vi "Eurotherm_Hardware_Module.vi"(3 "SP":bool=TRUE, 4 "Decimales":u16(ring)=1 items=["0"=1, "1"=10, "2"=100], 5 "Eurotherm (T:Enable)":bool=TRUE, 7 "Command":T2, 8 "error in (no error)":errorcluster, 9 "Value":dbl format="%04.1g", 10 "Address":T1(ring), 11 "VISA resource name":refnum<visa-resource-name>) -> (0 "error out":errorcluster, 1 "PV(C)":dbl, 2 "SP(C)":dbl)   [LabVIEW 2013]
uses:
  Eurotherm_Hardware_Module Control.ctl
  <vilib>/Instr/_visa.llb/VISA Configure Serial Port (Instr).vi
panel:
  out "String Read":string
  out "String Write":string
  # "Input Data"
  # "Local Data"
  # "Output Data"
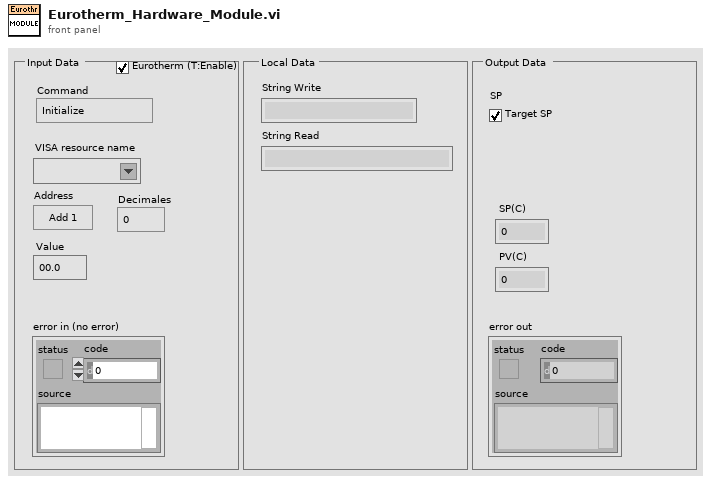
[diagram p1: front panel]
types:
  T1 = enum16{"Add 1", "Add 2", "Add 10", "Add 11", "Add 12", "Add 13"}
  T2 = typedef "Eurotherm_Hardware_Module Control.ctl" = enum16{"Initialize", "Write SP", "Read SP+PV", "Write Rate", "Set P", "Set I", "Set D", "Shutdown"}
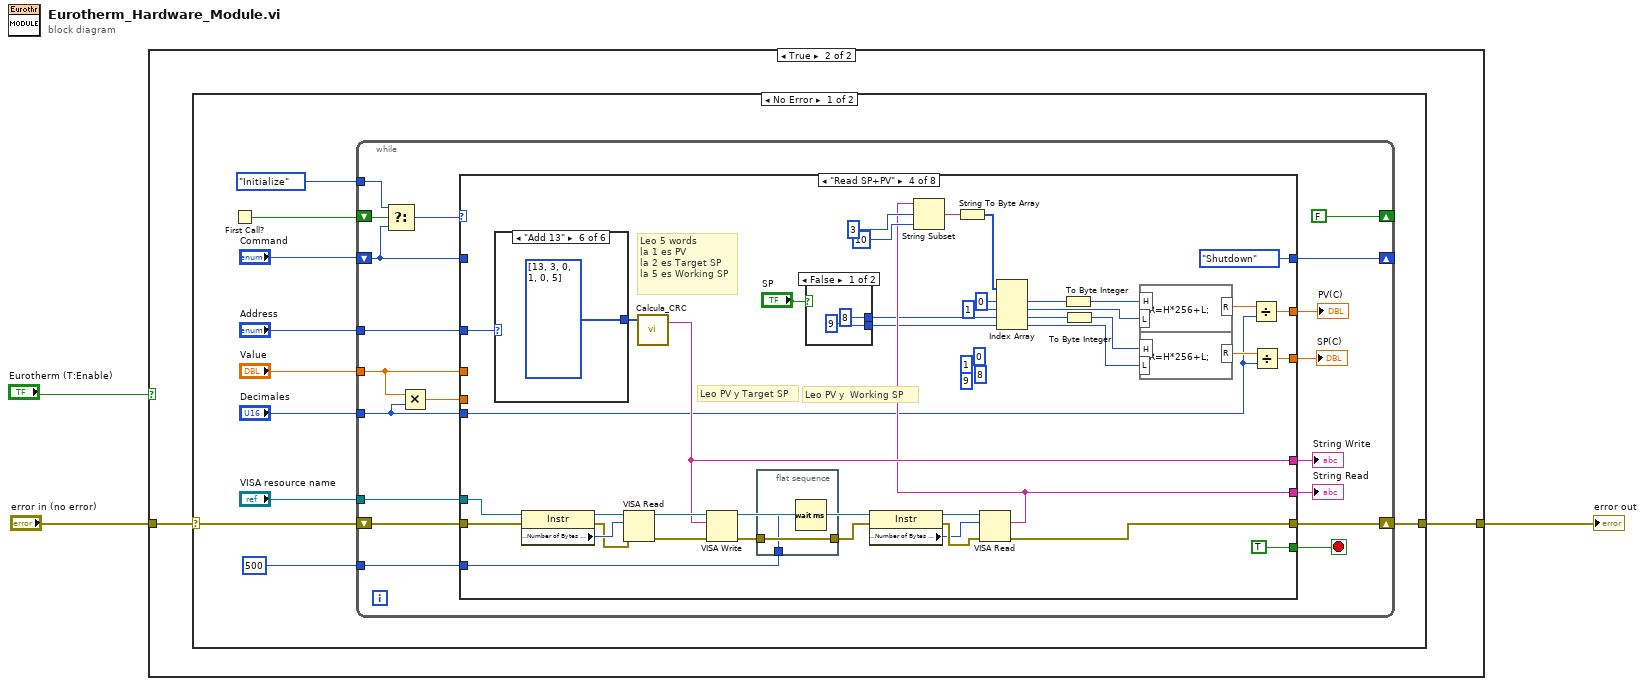
[diagram p0: block diagram]
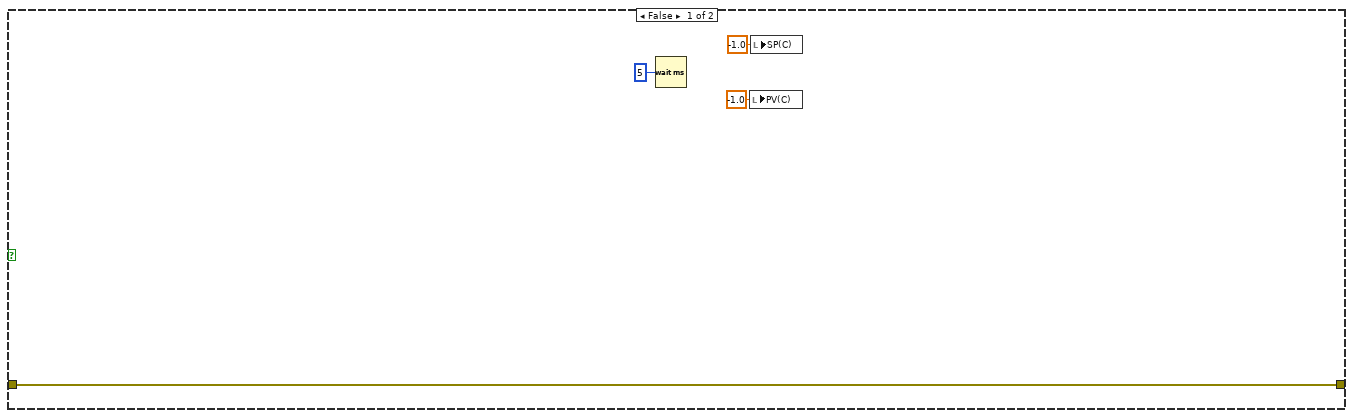
[diagram p2: hidden frame]
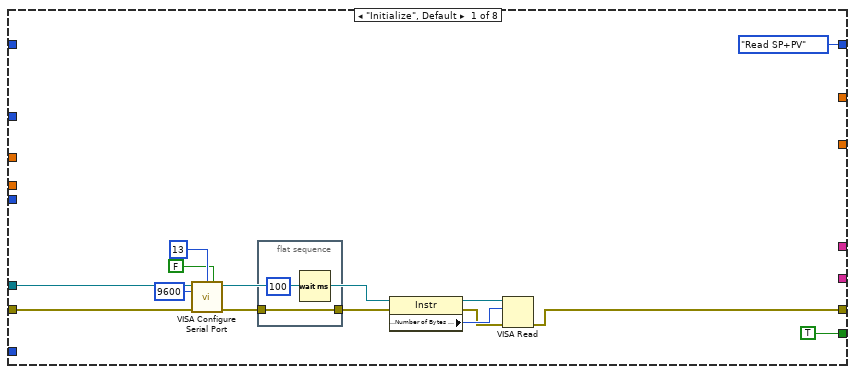
[diagram p3: hidden frame]
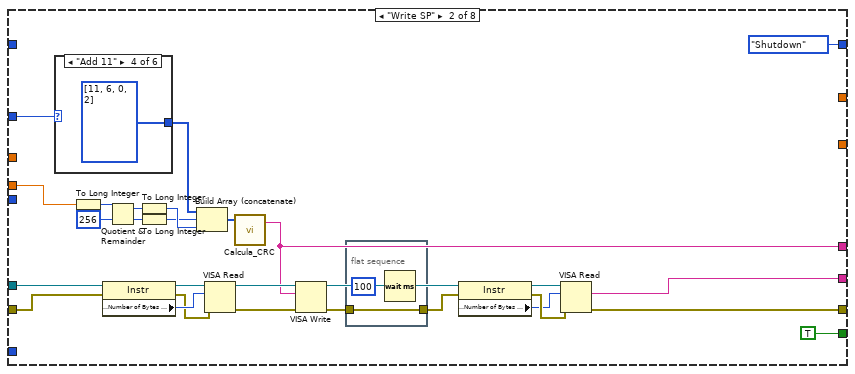
[diagram p4: hidden frame]
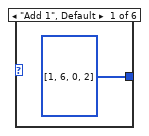
[diagram p5: hidden frame]
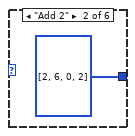
[diagram p6: hidden frame]
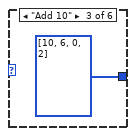
[diagram p7: hidden frame]
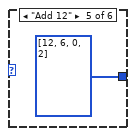
[diagram p8: hidden frame]
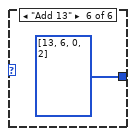
[diagram p9: hidden frame]
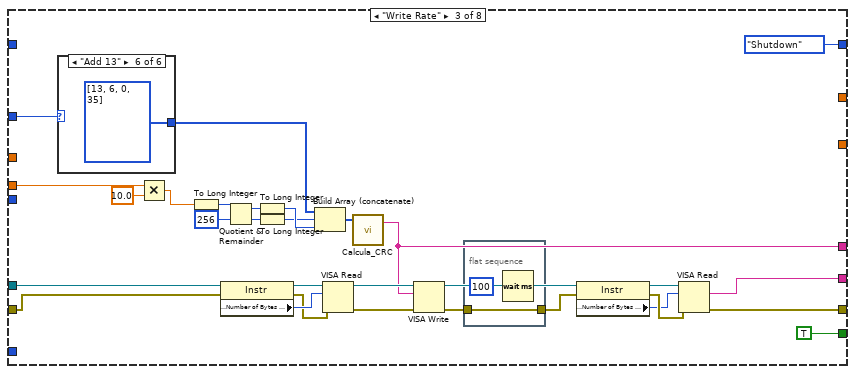
[diagram p10: hidden frame]
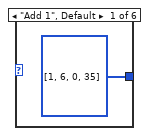
[diagram p11: hidden frame]
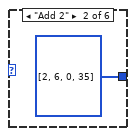
[diagram p12: hidden frame]
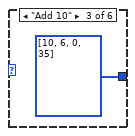
[diagram p13: hidden frame]
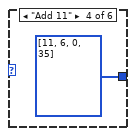
[diagram p14: hidden frame]
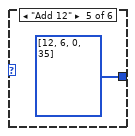
[diagram p15: hidden frame]
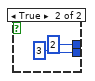
[diagram p16: hidden frame]
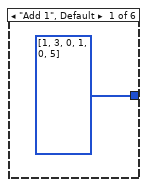
[diagram p17: hidden frame]
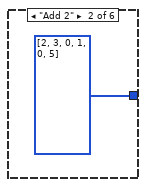
[diagram p18: hidden frame]
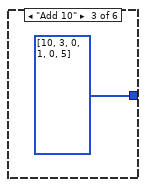
[diagram p19: hidden frame]
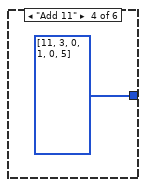
[diagram p20: hidden frame]
diagram:
  n1 = case shown="True" "Eurotherm (T:Enable)" {
    tunnel: "error in (no error)" -> [w7 w9]
    tunnel: [w7 w8] -> w2
    frame False {
      n2 = Wait (ms)(milliseconds to wait=u32 5) -> ()  [unwired: 1 out]
      n3 = local write "PV(C)"(-1.0 ("PV(C)")) -> ()
      n4 = local write "SP(C)"(-1.0 ("SP(C)")) -> ()
    }
    frame True {
      n5 = case shown="No Error" w9 {
        selector: w9 -> [w17 w295]
        tunnel: [w16 w295] -> w8
        frame No Error {
          n6 = First Call?() -> (First Call?: T/F=w19:bool)
          n7 = while {
            shift-right: [w33] -> _
            shift-left: "Command" -> [w34]
            shift-right: [w31] -> w16
            shift-left: w17 -> [w30]
            shift-right: [FALSE ("First Call?: T/F")] -> _
            shift-left: w19 -> [w38]
            tunnel: Eurotherm_Hardware_Module_Control."Initialize" ("t") -> [w37]
            tunnel: "Address" -> [w27]
            tunnel: "Value" -> [w22]
            tunnel: "Decimales" -> [w24]
            tunnel: "VISA resource name" -> [w21]
            tunnel: u32 500 ("milliseconds to wait") -> [w20]
            stop <- w32 stop-if-true
            n8 = Select(t=w37, s=w38, f=w34) -> (s? t:f=w35:T2)
            n9 = Multiply(x=w22, y=w24) -> (x*y=w23:dbl)
            n10 = case shown="\"Read SP+PV\"" w35 {
              tunnel: w34 -> [_ _ _ _ _ _ _ _]
              tunnel: [Eurotherm_Hardware_Module_Control."Read SP+PV" ("s? t:f") Eurotherm_Hardware_Module_Control."Shutdown" ("s? t:f") Eurotherm_Hardware_Module_Control."Shutdown" ("s? t:f") Eurotherm_Hardware_Module_Control."Shutdown" ("s? t:f") Eurotherm_Hardware_Module_Control."Shutdown" ("s? t:f") Eurotherm_Hardware_Module_Control."Shutdown" ("s? t:f") Eurotherm_Hardware_Module_Control."Shutdown" ("s? t:f") Eurotherm_Hardware_Module_Control."Shutdown" ("s? t:f")] -> w33
              tunnel: [TRUE ("First Call?: T/F") TRUE ("First Call?: T/F") TRUE ("First Call?: T/F") TRUE ("First Call?: T/F") TRUE ("First Call?: T/F") TRUE ("First Call?: T/F") TRUE ("First Call?: T/F") TRUE ("First Call?: T/F")] -> w32
              tunnel: [w42 w62 w96 w140 w189 w225 w261 w290] -> w31
              tunnel: w30 -> [w43 w63 w100 w156 w190 w226 w262 w291]
              tunnel: w21 -> [w39 w61 w101 w155 w188 w224 w260 w292]
              tunnel: [_ w60 w95 w141 w187 w223 w259 _] -> w29
              tunnel: [_ w59 w94 w154 w186 w222 w258 _] -> w28
              tunnel: w27 -> [_ w56 w99 w169 w183 w219 w255 _]
              tunnel: [_ _ _ w136 _ _ _ _] -> w26
              tunnel: [_ _ _ w135 _ _ _ _] -> w25
              tunnel: w23 -> [_ w55 w93 _ _ _ _ _]
              tunnel: w24 -> [_ _ _ w137 _ _ _ _]
              tunnel: w22 -> [_ _ _ _ w182 w218 w254 _]
              tunnel: w20 -> [_ _ _ w132 _ _ _ _]
              frame "Initialize", Default {
                n11 = call-poly "VISA Configure Serial Port"("VISA resource name"=w39, "termination char\n(0xA = '\\n' = LF)"=u8 13 ("termination char\n(0xA = '\\n' = LF)"), "Enable Termination\nChar (T)"=FALSE ("Enable Termination\nChar (T)"), "baud rate (9600)"=u32 9600, "error in (no error)"=w43) -> ("VISA resource name out"=w44:refnum<visa-resource-name>, "error out"=w45:errorcluster)  [unwired: 9 in]
                n12 = flat-sequence {
                  tunnel: w45 -> [w53]
                  tunnel: [w53] -> w52
                  frame #0 {
                    n13 = Wait (ms)(milliseconds to wait=u32 100) -> ()  [unwired: 1 out]
                  }
                }
                n14 = property class="Instr"(reference=w44, error in=w52) -> (reference out=w49:refnum<visa-resource-name>, error out=w50:errorcluster, "Serial Settings:Number of Bytes at Serial Port"=w51:u32)
                n15 = VISA Read(VISA resource name=w49, byte count=w51, error in (no error)=w50) -> (error out=w42:errorcluster)  [unwired: 3 out]
              }
              frame "Write SP" {
                n16 = case shown="\"Add 11\"" w56 {
                  tunnel: [u8[] [1, 6, 0, 2] ("Message Data") u8[] [2, 6, 0, 2] ("Message Data") u8[] [10, 6, 0, 2] ("Message Data") u8[] [11, 6, 0, 2] ("Message Data") u8[] [12, 6, 0, 2] ("Message Data") u8[] [13, 6, 0, 2] ("Message Data")] -> w82
                  frame "Add 1", Default {
                  }
                  frame "Add 2" {
                  }
                  frame "Add 10" {
                  }
                  frame "Add 11" {
                  }
                  frame "Add 12" {
                  }
                  frame "Add 13" {
                  }
                }
                n17 = To Long Integer(number=w55) -> (32bit integer=w81:i32)
                n18 = property class="Instr"(reference=w61, error in=w63) -> (reference out=w64:refnum<visa-resource-name>, error out=w65:errorcluster, "Serial Settings:Number of Bytes at Serial Port"=w66:u32)
                n19 = Quotient & Remainder(x=w81, y=256) -> (x-y*floor(x/y)=w76:i32, floor(x/y)=w77:i32)
                n20 = To Long Integer(number=w76) -> (32bit integer=w79:i32)
                n21 = To Long Integer(number=w77) -> (32bit integer=w78:i32)
                n22 = Build Array (concatenate)(w82, w78, w79) -> (w80:i32[])
                n23 = VISA Read(VISA resource name=w64, byte count=w66, error in (no error)=w65) -> (VISA resource name out=w73:refnum<visa-resource-name>, error out=w72:errorcluster)  [unwired: 2 out]
                n24 = call "Calcula_CRC.vi"("Message Data"=w80) -> ("String"=w59:string)  [unwired: 2 in, 1 out]
                n25 = VISA Write(VISA resource name=w73, write buffer=w59, error in (no error)=w72) -> (VISA resource name out=w74:refnum<visa-resource-name>, error out=w71:errorcluster)  [unwired: 1 out]
                n26 = flat-sequence {
                  tunnel: w71 -> [w83]
                  tunnel: [w83] -> w70
                  frame #0 {
                    n27 = Wait (ms)(milliseconds to wait=u32 100) -> ()  [unwired: 1 out]
                  }
                }
                n28 = property class="Instr"(reference=w74, error in=w70) -> (reference out=w69:refnum<visa-resource-name>, error out=w68:errorcluster, "Serial Settings:Number of Bytes at Serial Port"=w67:u32)
                n29 = VISA Read(VISA resource name=w69, byte count=w67, error in (no error)=w68) -> (read buffer=w60:string, error out=w62:errorcluster)  [unwired: 2 out]
              }
              frame "Write Rate" {
                n30 = case shown="\"Add 13\"" w99 {
                  tunnel: [u8[] [1, 6, 0, 35] ("Message Data") u8[] [2, 6, 0, 35] ("Message Data") u8[] [10, 6, 0, 35] ("Message Data") u8[] [11, 6, 0, 35] ("Message Data") u8[] [12, 6, 0, 35] ("Message Data") u8[] [13, 6, 0, 35] ("Message Data")] -> w120
                  frame "Add 1", Default {
                  }
                  frame "Add 2" {
                  }
                  frame "Add 10" {
                  }
                  frame "Add 11" {
                  }
                  frame "Add 12" {
                  }
                  frame "Add 13" {
                  }
                }
                n31 = Multiply(x=w93, y=10.0) -> (x*y=w92:dbl)
                n32 = To Long Integer(number=w92) -> (32bit integer=w119:i32)
                n33 = property class="Instr"(reference=w101, error in=w100) -> (reference out=w102:refnum<visa-resource-name>, error out=w103:errorcluster, "Serial Settings:Number of Bytes at Serial Port"=w104:u32)
                n34 = Quotient & Remainder(x=w119, y=256) -> (x-y*floor(x/y)=w114:i32, floor(x/y)=w115:i32)
                n35 = To Long Integer(number=w114) -> (32bit integer=w117:i32)
                n36 = To Long Integer(number=w115) -> (32bit integer=w116:i32)
                n37 = Build Array (concatenate)(w120, w116, w117) -> (w118:i32[])
                n38 = VISA Read(VISA resource name=w102, byte count=w104, error in (no error)=w103) -> (VISA resource name out=w111:refnum<visa-resource-name>, error out=w110:errorcluster)  [unwired: 2 out]
                n39 = call "Calcula_CRC.vi"("Message Data"=w118) -> ("String"=w94:string)  [unwired: 2 in, 1 out]
                n40 = VISA Write(VISA resource name=w111, write buffer=w94, error in (no error)=w110) -> (VISA resource name out=w112:refnum<visa-resource-name>, error out=w109:errorcluster)  [unwired: 1 out]
                n41 = flat-sequence {
                  tunnel: w109 -> [w121]
                  tunnel: [w121] -> w108
                  frame #0 {
                    n42 = Wait (ms)(milliseconds to wait=u32 100) -> ()  [unwired: 1 out]
                  }
                }
                n43 = property class="Instr"(reference=w112, error in=w108) -> (reference out=w107:refnum<visa-resource-name>, error out=w106:errorcluster, "Serial Settings:Number of Bytes at Serial Port"=w105:u32)
                n44 = VISA Read(VISA resource name=w107, byte count=w105, error in (no error)=w106) -> (read buffer=w95:string, error out=w96:errorcluster)  [unwired: 2 out]
              }
              frame "Read SP+PV" {
                (unwired) 9 ("index")
                (unwired) 8 ("index")
                (unwired) 1 ("index")
                (unwired) 0 ("index")
                # "Leo PV y  Working SP"
                # "Leo PV y Target SP"
                # "Leo 5 words\nla 1 es PV\nla 2 es Target SP\nla 5 es Working SP"
                n45 = case shown="\"Add 13\"" w169 {
                  tunnel: [u8[] [1, 3, 0, 1, 0, 5] ("Message Data") u8[] [2, 3, 0, 1, 0, 5] ("Message Data") u8[] [10, 3, 0, 1, 0, 5] ("Message Data") u8[] [11, 3, 0, 1, 0, 5] ("Message Data") u8[] [12, 3, 0, 1, 0, 5] ("Message Data") u8[] [13, 3, 0, 1, 0, 5] ("Message Data")] -> w168
                  frame "Add 1", Default {
                  }
                  frame "Add 2" {
                  }
                  frame "Add 10" {
                  }
                  frame "Add 11" {
                  }
                  frame "Add 12" {
                  }
                  frame "Add 13" {
                  }
                }
                n46 = property class="Instr"(reference=w155, error in=w156) -> (reference out=w157:refnum<visa-resource-name>, error out=w158:errorcluster, "Serial Settings:Number of Bytes at Serial Port"=w159:u32)
                n47 = VISA Read(VISA resource name=w157, byte count=w159, error in (no error)=w158) -> (VISA resource name out=w166:refnum<visa-resource-name>, error out=w165:errorcluster)  [unwired: 2 out]
                n48 = call "Calcula_CRC.vi"("Message Data"=w168) -> ("String"=w154:string)  [unwired: 2 in, 1 out]
                n49 = VISA Write(VISA resource name=w166, write buffer=w154, error in (no error)=w165) -> (VISA resource name out=w167:refnum<visa-resource-name>, error out=w164:errorcluster)  [unwired: 1 out]
                n50 = flat-sequence {
                  tunnel: w164 -> [w175]
                  tunnel: [w175] -> w163
                  tunnel: w132 -> [w174]
                  frame #0 {
                    n51 = Wait (ms)(milliseconds to wait=w174) -> ()  [unwired: 1 out]
                  }
                }
                n52 = case shown="False" "SP" {
                  tunnel: [8 ("index") 2 ("index")] -> w130
                  tunnel: [9 ("index") 3 ("index")] -> w129
                  frame False {
                  }
                  frame True {
                  }
                }
                n53 = property class="Instr"(reference=w167, error in=w163) -> (reference out=w162:refnum<visa-resource-name>, error out=w161:errorcluster, "Serial Settings:Number of Bytes at Serial Port"=w160:u32)
                n54 = VISA Read(VISA resource name=w162, byte count=w160, error in (no error)=w161) -> (read buffer=w141:string, error out=w140:errorcluster)  [unwired: 2 out]
                n55 = String Subset(string=w141, offset (0)=3, length (rest)=10 ("length (rest)")) -> (substring=w146:string)
                n56 = String To Byte Array(string=w146) -> (unsigned byte array=w149:u8[])
                n57 = Index Array(array=w149, index #1=0 ("index"), index #2=1 ("index"), index #3=w130, index #4=w129) -> (element #1=w145:u8, element #2=w144:u8, element #3=w143:u8, element #4=w142:u8)
                n58 = To Byte Integer(number=w145) -> (8bit integer=w134:i8)
                n59 = To Byte Integer(number=w143) -> (8bit integer=w133:i8)
                n60 = formula code="R=H*256+L;"("H"=w134, "L"=w144) -> ("R"=w139:dbl)
                n61 = formula code="R=H*256+L;"("H"=w133, "L"=w142) -> ("R"=w138:dbl)
                n62 = Divide(x=w139, y=w137) -> (x/y=w136:dbl)
                n63 = Divide(x=w138, y=w137) -> (x/y=w135:dbl)
              }
              frame "Set P" {
                n64 = case shown="\"Add 1\", Default" w183 {
                  tunnel: [u8[] [1, 6, 0, 6] ("Message Data") u8[] [2, 6, 0, 6] ("Message Data") u8[] [10, 6, 0, 6] ("Message Data") u8[] [11, 6, 0, 6] ("Message Data") u8[] [12, 6, 0, 6] ("Message Data") u8[] [13, 6, 0, 6] ("Message Data")] -> w209
                  frame "Add 1", Default {
                  }
                  frame "Add 2" {
                  }
                  frame "Add 10" {
                  }
                  frame "Add 11" {
                  }
                  frame "Add 12" {
                  }
                  frame "Add 13" {
                  }
                }
                n65 = To Long Integer(number=w182) -> (32bit integer=w208:i32)
                n66 = property class="Instr"(reference=w188, error in=w190) -> (reference out=w191:refnum<visa-resource-name>, error out=w192:errorcluster, "Serial Settings:Number of Bytes at Serial Port"=w193:u32)
                n67 = Quotient & Remainder(x=w208, y=256) -> (x-y*floor(x/y)=w203:i32, floor(x/y)=w204:i32)
                n68 = To Long Integer(number=w203) -> (32bit integer=w206:i32)
                n69 = To Long Integer(number=w204) -> (32bit integer=w205:i32)
                n70 = Build Array (concatenate)(w209, w205, w206) -> (w207:i32[])
                n71 = VISA Read(VISA resource name=w191, byte count=w193, error in (no error)=w192) -> (VISA resource name out=w200:refnum<visa-resource-name>, error out=w199:errorcluster)  [unwired: 2 out]
                n72 = call "Calcula_CRC.vi"("Message Data"=w207) -> ("String"=w186:string)  [unwired: 2 in, 1 out]
                n73 = VISA Write(VISA resource name=w200, write buffer=w186, error in (no error)=w199) -> (VISA resource name out=w201:refnum<visa-resource-name>, error out=w198:errorcluster)  [unwired: 1 out]
                n74 = flat-sequence {
                  tunnel: w198 -> [w210]
                  tunnel: [w210] -> w197
                  frame #0 {
                    n75 = Wait (ms)(milliseconds to wait=u32 100) -> ()  [unwired: 1 out]
                  }
                }
                n76 = property class="Instr"(reference=w201, error in=w197) -> (reference out=w196:refnum<visa-resource-name>, error out=w195:errorcluster, "Serial Settings:Number of Bytes at Serial Port"=w194:u32)
                n77 = VISA Read(VISA resource name=w196, byte count=w194, error in (no error)=w195) -> (read buffer=w187:string, error out=w189:errorcluster)  [unwired: 2 out]
              }
              frame "Set I" {
                n78 = case shown="\"Add 13\"" w219 {
                  tunnel: [u8[] [1, 6, 0, 8] ("Message Data") u8[] [2, 6, 0, 8] ("Message Data") u8[] [10, 6, 0, 8] ("Message Data") u8[] [11, 6, 0, 8] ("Message Data") u8[] [12, 6, 0, 8] ("Message Data") u8[] [13, 6, 0, 8] ("Message Data")] -> w245
                  frame "Add 1", Default {
                  }
                  frame "Add 2" {
                  }
                  frame "Add 10" {
                  }
                  frame "Add 11" {
                  }
                  frame "Add 12" {
                  }
                  frame "Add 13" {
                  }
                }
                n79 = To Long Integer(number=w218) -> (32bit integer=w244:i32)
                n80 = property class="Instr"(reference=w224, error in=w226) -> (reference out=w227:refnum<visa-resource-name>, error out=w228:errorcluster, "Serial Settings:Number of Bytes at Serial Port"=w229:u32)
                n81 = Quotient & Remainder(x=w244, y=256) -> (x-y*floor(x/y)=w239:i32, floor(x/y)=w240:i32)
                n82 = To Long Integer(number=w239) -> (32bit integer=w242:i32)
                n83 = To Long Integer(number=w240) -> (32bit integer=w241:i32)
                n84 = Build Array (concatenate)(w245, w241, w242) -> (w243:i32[])
                n85 = VISA Read(VISA resource name=w227, byte count=w229, error in (no error)=w228) -> (VISA resource name out=w236:refnum<visa-resource-name>, error out=w235:errorcluster)  [unwired: 2 out]
                n86 = call "Calcula_CRC.vi"("Message Data"=w243) -> ("String"=w222:string)  [unwired: 2 in, 1 out]
                n87 = VISA Write(VISA resource name=w236, write buffer=w222, error in (no error)=w235) -> (VISA resource name out=w237:refnum<visa-resource-name>, error out=w234:errorcluster)  [unwired: 1 out]
                n88 = flat-sequence {
                  tunnel: w234 -> [w246]
                  tunnel: [w246] -> w233
                  frame #0 {
                    n89 = Wait (ms)(milliseconds to wait=u32 100) -> ()  [unwired: 1 out]
                  }
                }
                n90 = property class="Instr"(reference=w237, error in=w233) -> (reference out=w232:refnum<visa-resource-name>, error out=w231:errorcluster, "Serial Settings:Number of Bytes at Serial Port"=w230:u32)
                n91 = VISA Read(VISA resource name=w232, byte count=w230, error in (no error)=w231) -> (read buffer=w223:string, error out=w225:errorcluster)  [unwired: 2 out]
              }
              frame "Set D" {
                n92 = case shown="\"Add 13\"" w255 {
                  tunnel: [u8[] [1, 6, 0, 9] ("Message Data") u8[] [2, 6, 0, 9] ("Message Data") u8[] [10, 6, 0, 9] ("Message Data") u8[] [11, 6, 0, 9] ("Message Data") u8[] [12, 6, 0, 9] ("Message Data") u8[] [13, 6, 0, 9] ("Message Data")] -> w281
                  frame "Add 1", Default {
                  }
                  frame "Add 2" {
                  }
                  frame "Add 10" {
                  }
                  frame "Add 11" {
                  }
                  frame "Add 12" {
                  }
                  frame "Add 13" {
                  }
                }
                n93 = To Long Integer(number=w254) -> (32bit integer=w280:i32)
                n94 = property class="Instr"(reference=w260, error in=w262) -> (reference out=w263:refnum<visa-resource-name>, error out=w264:errorcluster, "Serial Settings:Number of Bytes at Serial Port"=w265:u32)
                n95 = Quotient & Remainder(x=w280, y=256) -> (x-y*floor(x/y)=w275:i32, floor(x/y)=w276:i32)
                n96 = To Long Integer(number=w275) -> (32bit integer=w278:i32)
                n97 = To Long Integer(number=w276) -> (32bit integer=w277:i32)
                n98 = Build Array (concatenate)(w281, w277, w278) -> (w279:i32[])
                n99 = VISA Read(VISA resource name=w263, byte count=w265, error in (no error)=w264) -> (VISA resource name out=w272:refnum<visa-resource-name>, error out=w271:errorcluster)  [unwired: 2 out]
                n100 = call "Calcula_CRC.vi"("Message Data"=w279) -> ("String"=w258:string)  [unwired: 2 in, 1 out]
                n101 = VISA Write(VISA resource name=w272, write buffer=w258, error in (no error)=w271) -> (VISA resource name out=w273:refnum<visa-resource-name>, error out=w270:errorcluster)  [unwired: 1 out]
                n102 = flat-sequence {
                  tunnel: w270 -> [w282]
                  tunnel: [w282] -> w269
                  frame #0 {
                    n103 = Wait (ms)(milliseconds to wait=u32 100) -> ()  [unwired: 1 out]
                  }
                }
                n104 = property class="Instr"(reference=w273, error in=w269) -> (reference out=w268:refnum<visa-resource-name>, error out=w267:errorcluster, "Serial Settings:Number of Bytes at Serial Port"=w266:u32)
                n105 = VISA Read(VISA resource name=w268, byte count=w266, error in (no error)=w267) -> (read buffer=w259:string, error out=w261:errorcluster)  [unwired: 2 out]
              }
              frame "Shutdown" {
                n106 = VISA Close(VISA resource name=w292, error in (no error)=w291) -> (error out=w290:errorcluster)
              }
            }
            "String Read" <- w29
            "String Write" <- w28
            "SP(C)" <- w25
            "PV(C)" <- w26
          }
        }
        frame Error {
        }
      }
    }
  }
  "error out" <- w2
